vi "Calculate Multi Points Kb.vi"(8 "error in (no error)":errorcluster, 11 "Calibration 2D Table":dbl[][](array[numeric])) -> (0 "error out":errorcluster, 3 "Calibration":T1)   [LabVIEW 2015, in "SQLite.lvclass"]
uses:
  SQLite.lvclass
  Calibration Kb and Volt.ctl
  Calibration K and b Array.ctl
  Calibration K and b.ctl
  <userlib>/_MGI/1D Array/MGI Calculate Array Differences/MGI Calculate Array Differences (DBL[]).vi
panel:
  out "x/y":dbl[](array[numeric])
  out "y(i)=x(i)-x(i-1)":dbl[](array[numeric]) format="%.2f"
  out "y(i)=x(i)-x(i-1) 2":dbl[](array[numeric]) format="%.2f"
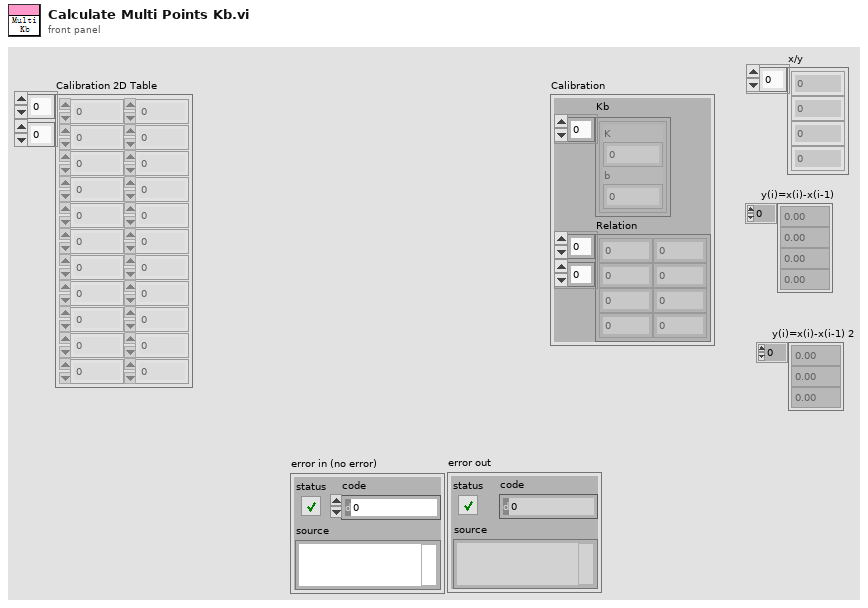
[diagram p1: front panel]
types:
  T1 = typedef "SQLite.lvclass/Calibration Kb and Volt.ctl" = cluster{"Kb":T2, "Relation":dbl[][]}
  T2 = typedef "SQLite.lvclass/Calibration K and b Array.ctl" = T3[]
  T3 = typedef "SQLite.lvclass/Calibration K and b.ctl" = cluster{"K":dbl, "b":dbl}
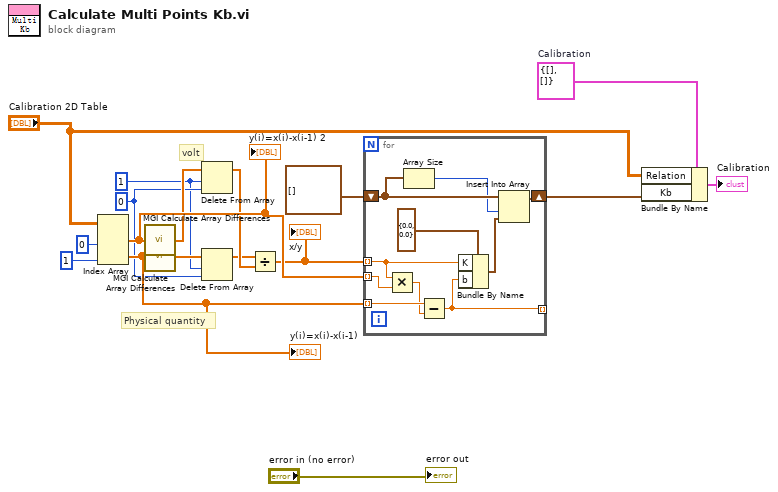
[diagram p0: block diagram]
diagram:
  w3 = T1 {"Kb"=[], "Relation"=[]}  # Calibration
  w8 = 0 ("index")
  w7 = 1 ("length")
  # "Physical quantity"
  # "volt"
  n1 = Index Array(array="Calibration 2D Table", index (col) #1=0 ("disabled index (col)"), index (col) #2=1 ("index (col)")) -> (element #1=w14:dbl[], element #2=w15:dbl[])  [unwired: 2 in]
  "y(i)=x(i)-x(i-1)" <- w15
  "y(i)=x(i)-x(i-1) 2" <- w14
  n2 = call-poly <userlib>:"MGI Calculate Array Differences.vi"("x(i)"=w14) -> ("y(i)=x(i)-x(i-1)"=w12:dbl[])  [unwired: 1 in]
  n3 = call-poly <userlib>:"MGI Calculate Array Differences.vi"("x(i)"=w15) -> ("y(i)=x(i)-x(i-1)"=w16:dbl[])  [unwired: 1 in]
  n4 = Delete From Array(array=w12, length=w7, index=w8) -> (array with subset deleted=w10:dbl[])  [unwired: 1 out]
  n5 = Delete From Array(array=w16, length=w7, index=w8) -> (array with subset deleted=w9:dbl[])  [unwired: 1 out]
  n6 = Divide(x=w9, y=w10) -> (x/y=w11:dbl[])
  "x/y" <- w11
  n7 = for {
    tunnel: w11 -> [w24] mode=indexing
    tunnel: w14 -> [w27] mode=indexing
    tunnel: w15 -> [w26] mode=indexing
    tunnel: [w23] -> _ mode=indexing
    shift-right: [w22] -> w13
    shift-left: T2 [] ("Kb Array") -> [w21]
    n8 = Multiply(x=w24, y=w27) -> (x*y=w25:dbl)
    n9 = Array Size(array=w21) -> (size(s)=w20:i32)
    n10 = Subtract(x=w26, y=w25) -> (x-y=w23:dbl)
    n11 = Bundle By Name(cluster=T3 {"K"=0.0, "b"=0.0} ("Calibration"), "K"=w24, "b"=w23) -> (w19:T3)
    n12 = Insert Into Array(array=w21, index=w20, new element=w19) -> (w22:T2)
  }
  n13 = Bundle By Name(cluster=w3, "Relation"="Calibration 2D Table", "Kb"=w13) -> (→"Calibration":T1)
  "error out" <- "error in (no error)"
